vi "OnTextChange.vi"(0 "XRef":T11, 1 "ID":T10, 2 "Data":T10, 3 "State In":T1) -> (14 "Reply":T9, 15 "Fatal Error Out":T8, 16 "State Out":T1)   [LabVIEW 2020, in "Parallel Diagram Block.xnode"]
uses:
  Parallel Diagram Block.xnode
  <vilib>/XNodeSupport/XNodeString.ctl
  <vilib>/XNodeSupport/NI_XNodeSupport.lvlib
  <vilib>/XNodeSupport/XNodeStringArray.ctl
  Parallel Block/Direction.ctl
  Parallel Block/Parallel Block.lvlib
  <vilib>/XNodeSupport/XNodeXNodeRef.ctl
  <vilib>/XNodeSupport/XNodeErrorCluster.ctl
  State.ctl
  Parallel Block/Value Type.ctl
  Parallel Block/Type Descriptor.ctl
  <vilib>/picture/picture.llb/imagedata.ctl
  Parallel Block/Terminal Mode.ctl
  Parallel Block/Terminal Type.ctl
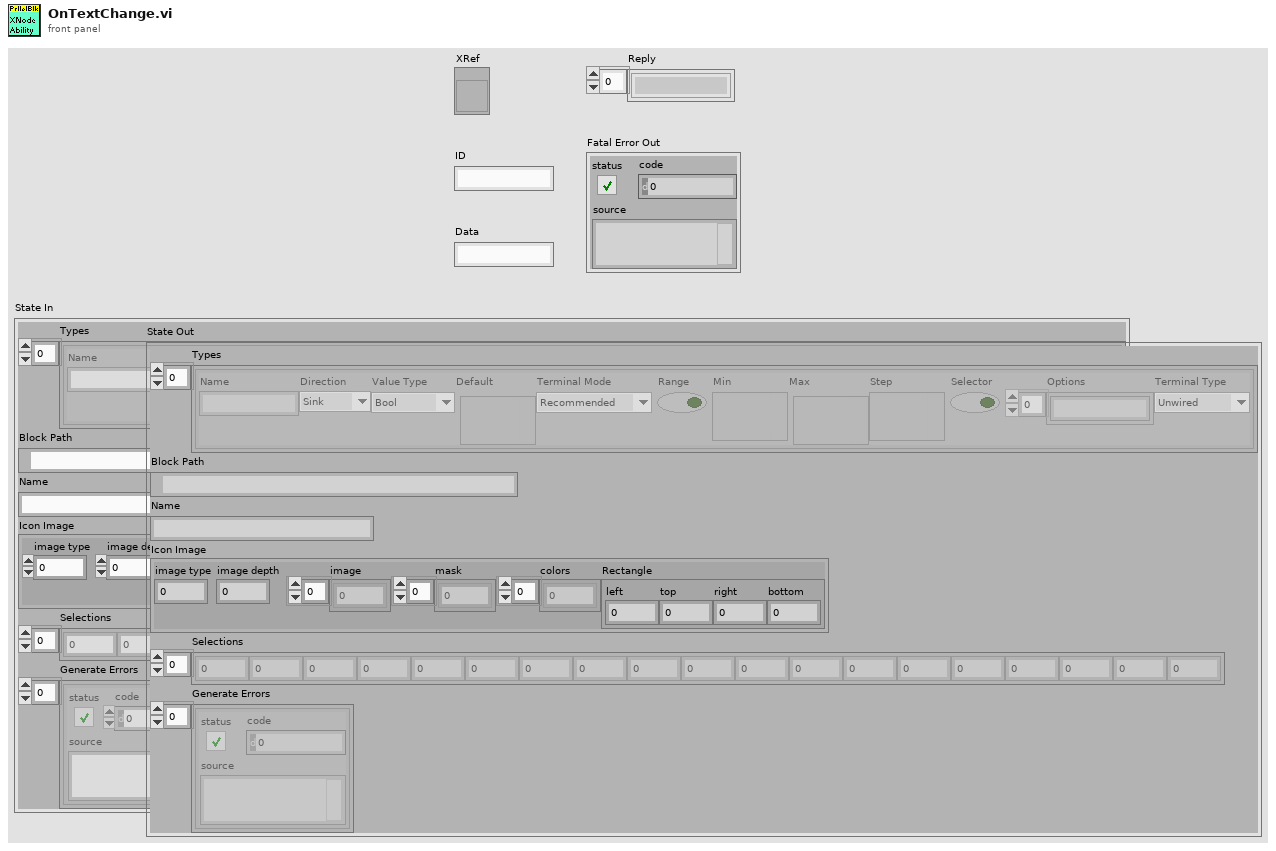
[diagram p1: front panel]
types:
  T1 = typedef "Parallel Diagram Block.xnode/State.ctl" = cluster{"Types":T2[], "Block Path":path, "Name":string, "Icon Image":T7, "Selections":i32[], "Generate Errors":errorcluster[]}
  T2 = typedef "Parallel Block.lvlib/Type Descriptor.ctl" = cluster{"Name":string, "Direction":T3, "Value Type":T4, "Default":variant, "Terminal Mode":T5, "Range":bool, "Min":variant, "Max":variant, "Step":variant, "Selector":bool, "Options":string[], "Terminal Type":T6}
  T3 = typedef "Parallel Block.lvlib/Direction.ctl" = enum16{"Sink", "Source"}
  T4 = typedef "Parallel Block.lvlib/Value Type.ctl" = enum16{"Unknown", "Bool", "U8", "U16", "U32", "U64", "I8", "I16", "I32", "I64", "SGL", "DBL", "CSG", "CDB", "CDBWfm", "String", "DBLWfm"}
  T5 = typedef "Parallel Block.lvlib/Terminal Mode.ctl" = enum16{"Recommended", "Required", "None"}
  T6 = typedef "Parallel Block.lvlib/Terminal Type.ctl" = enum16{"Unwired", "Connection", "Value", "Control Ref"}
  T7 = typedef "imagedata.ctl" = cluster{"image type":i32, "image depth":i32, "image":u8[], "mask":u8[], "colors":u32[], "Rectangle":cluster{"left":i16, "top":i16, "right":i16, "bottom":i16}}
  T8 = typedef "NI_XNodeSupport.lvlib/XNodeErrorCluster.ctl" = errorcluster
  T9 = typedef "NI_XNodeSupport.lvlib/XNodeStringArray.ctl" = T10[]
  T10 = typedef "NI_XNodeSupport.lvlib/XNodeString.ctl" = string
  T11 = typedef "NI_XNodeSupport.lvlib/XNodeXNodeRef.ctl" = refnum<vi>
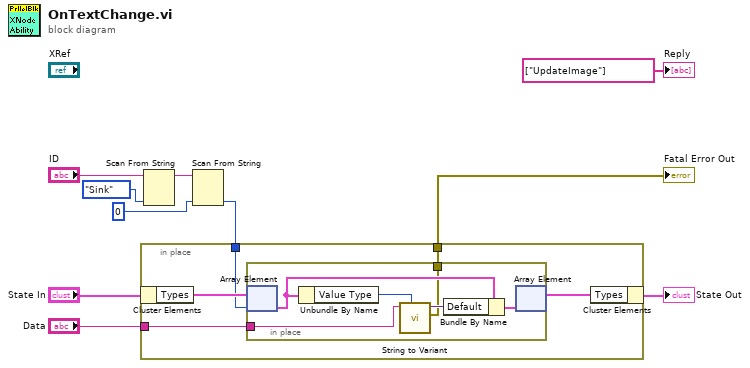
[diagram p0: block diagram]
diagram:
  n1 = Scan From String(input string="ID", default 1=Direction."Sink" ("Direction")) -> (remaining string=w8:string)  [unwired: 4 in, 2 out]
  n2 = Scan From String(input string=w8, default 1=0) -> (output 1=w5:i32)  [unwired: 3 in, 3 out]
  n3 = in-place {
    in-place-border: w5 -> [w13]
    in-place-border: "Data" -> [w12]
    in-place-border: [w11] -> w1
    n4 = in-place-cluster #1("State In") -> ("Types"=w15:T2[])
    n5 = in-place {
      in-place-border: w12 -> [w17]
      in-place-border: [w16] -> w11
      n6 = in-place-array #2(w15, w13) -> (w21:T2)
      n7 = Unbundle By Name(w21) -> ("Value Type"=w20:T4)
      n8 = call "String to Variant.vi"("Value Type"=w20, "String"=w17) -> ("error out"=w16:errorcluster, "Variant"=w19:variant)  [unwired: 8 in]
      n9 = Bundle By Name(cluster=w21, "Default"=w19) -> (w18:T2)
      n10 = in-place-array #2(w18) -> (w14:T2[])  [unwired: 1 out]
    }
    n11 = in-place-cluster #1("Types"=w14) -> (→"State Out":T1)
  }
  "Fatal Error Out" <- w1
  "Reply" <- T9 ["UpdateImage"] ("Reply")
